vi "FdxCmdMonQueueTellCvi.vi"(8 "error in":errorcluster, 9 "QueueId":u32, 11 "InstrumentHandle_port":u32) -> (0 "error out":errorcluster, 1 "QueueTellOut":cluster{"Position":u32, "ByteOffset":u32}, 3 "InstrumentHandle_port":u32)   [LabVIEW 2020, in "AIM664LV.lvlib"]
doc: "This function gets the actual read index to the data queue where the next queue read will occur.\nThis function is only applicable if the capture control is set to single (non-continuous)."
uses:
  AIM664LV.lvlib
  AFDX_LibraryAdmin/FdxGlobalDllPath.vi
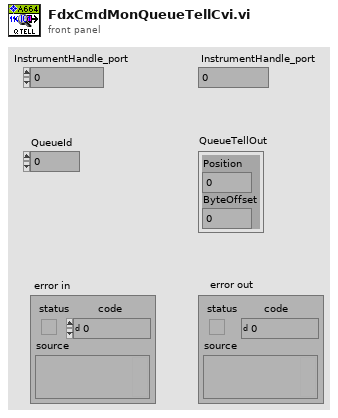
[diagram p1: front panel]
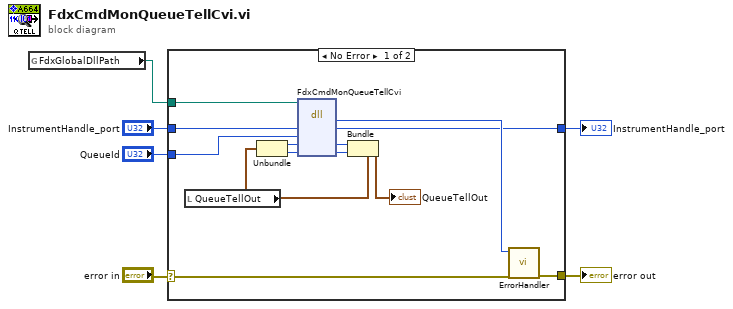
[diagram p0: block diagram]
diagram:
  n1 = global read "FdxGlobalDllPath.vi" "FdxGlobalDllPath"() -> (w4:path)
  n2 = case shown="No Error" "error in" {
    selector: "error in" -> [w18 w21]
    tunnel: [w19 w21] -> w6
    tunnel: w4 -> [w10 _]
    tunnel: [w9 w20] -> w3
    tunnel: "InstrumentHandle_port" -> [w8 w20]
    tunnel: "QueueId" -> [w7 _]
    frame No Error {
      n3 = local read "QueueTellOut"() -> (w11:cluster{"Position":u32, "ByteOffset":u32})
      n4 = Unbundle(w11) -> ("Position"=w12:u32, "ByteOffset"=w13:u32)
      n5 = dll-call lib="aim_fdx.19.dll" fn="FdxCmdMonQueueTellCvi"(path in=w10, "InstrumentHandle"=w8, "QueueId"=w7, "Position"=w12, "ByteOffset"=w13) -> ("status"=w17:i32, "InstrumentHandle"=w9:u32, "Position"=w15:u32, "ByteOffset"=w14:u32)  [unwired: 3 in, 2 out]
      n6 = Bundle(cluster=w11, "Position"=w15, "ByteOffset"=w14) -> (→"QueueTellOut":cluster{"Position":u32, "ByteOffset":u32})
      n7 = call "ErrorHandler.vi"("error in"=w18, "AIM Error"=w17) -> ("error out"=w19:errorcluster)  [unwired: 9 in]
    }
    frame Error {
    }
  }
  "error out" <- w6
  "InstrumentHandle_port" <- w3
